vi "Example_DIO_DWG_Array.vi"() -> ()   [LabVIEW 2013]
uses:
  <vilib>/Signadyne/Wave/base/newFromArrayInteger.vi
  <vilib>/Signadyne/Wave/base/waveformLoadWave.vi
  Instance          11 29Saved   Example_DIO_DWG_Array .vi
panel:
  in  "Data":i32[][](array[numeric])=[[0], [1], [2], [3], [4], [5], [6], [7], [8], [9], [10], [11], [12], [13], [14], [15], [16], [17], [18], [19], [20], [21], [22], [23], [24], [25], [26], [27], [28], [29], [30], [31]]
  in  "End Line":i32=19
  in  "Start Line":i32=16
  in  "Slot":i32=5
  out "ConfigBus Status":errorcluster
  out "DirConfig":errorcluster
  out "Bus value":i64
  out "Close Status":errorcluster
  in  "Stop Loop":bool
  out "Open Status":errorcluster
  in  "Part Number":string="SD-PXE-DIO-H0002"
  # "Output&Input Bus"
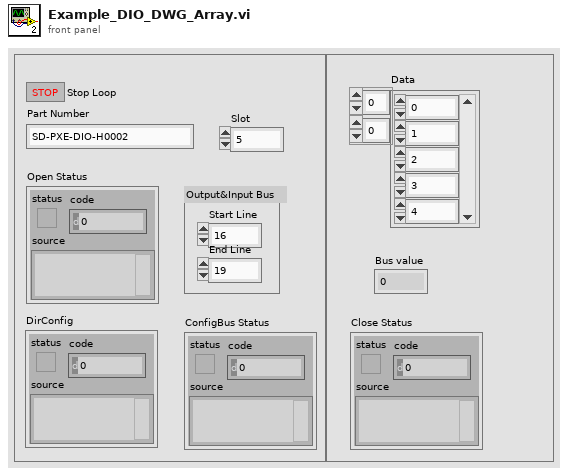
[diagram p1: front panel]
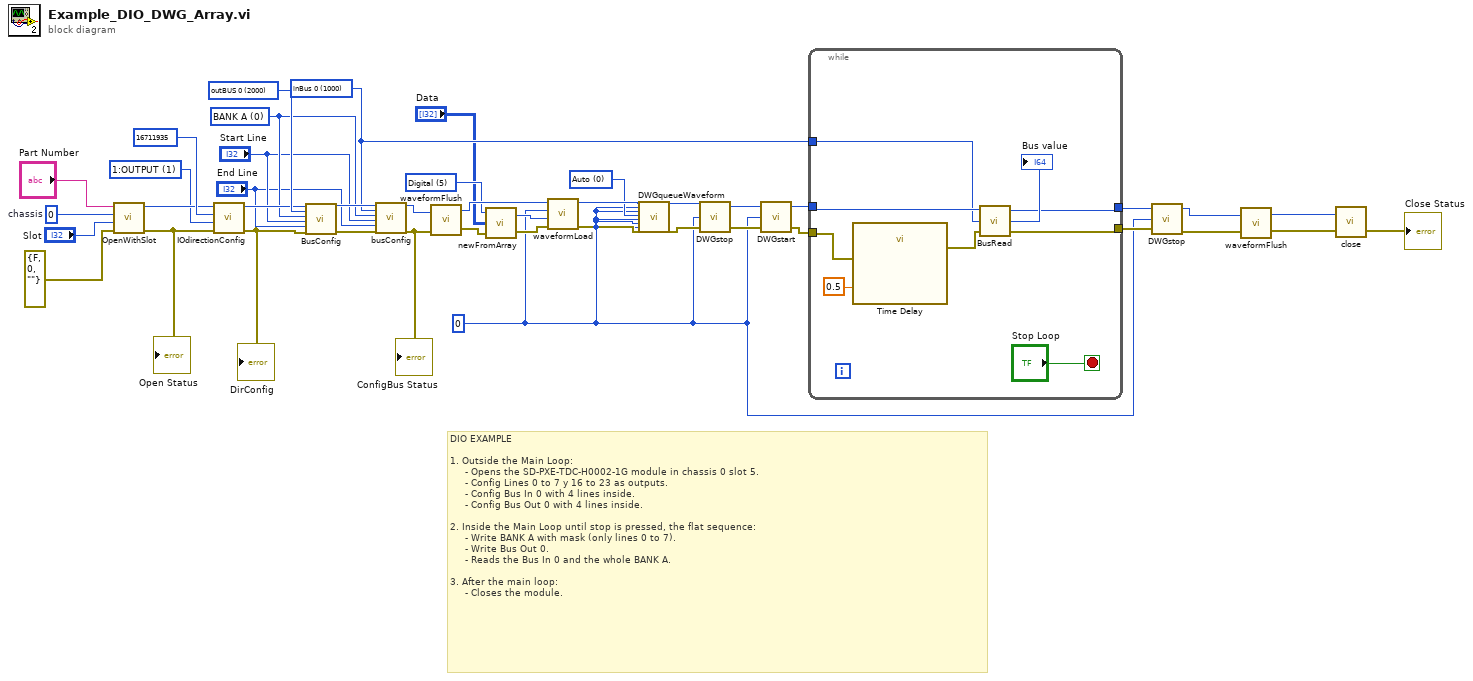
[diagram p0: block diagram]
diagram:
  w2 = 5 items=["Digital"=5] ("waveformType")
  w3 = 1000 items=["inBus 0"=1000, "inBus 1"=1001, "outBus 0"=2000, "outBus 1"=2001] ("nBus")
  w24 = 0 items=["Auto", "VI/HVI", "External"] ("triggerMode")
  w15 = 0 ("waveformNumber")
  w6 = 0 items=["BANK A"=0, "BANK B"=1, "BANK B:A"=3000] ("nPort")
  w35 = 2000 items=["inBus 0"=1000, "outBUS 0"=2000] ("nBus")
  w36 = u16 1 items=["0:INPUT", "1:OUTPUT"] ("direction")
  w40 = 0  # chassis
  # "DIO EXAMPLE\n\n1. Outside the Main Loop:\n     - Opens the SD-PXE-TDC-H0002-1G module in chassis 0 slot 5.\n     - Config Lines 0 to 7 y 16 to 23 as outputs.\n     - Config Bus In 0 with 4 lines inside.\n     - Config Bus Out 0 with 4 lines inside.\n\n2. Inside the Main Loop until stop is pressed, the flat sequence:\n     - Write BANK A with mask (only lines 0 to 7).\n     - Write Bus Out 0.\n     - Reads the Bus In 0 and the whole BANK A.\n\n3. After the main loop:\n     - Closes the module."
  n1 = call <vilib>:"OpenWithSlot.vi"("errorIn"=errorcluster {"status"=FALSE, "code"=0, "source"=""}, "nSlot"="Slot", "nChassis"=w40, "partNumber"="Part Number") -> ("errorOut"=w39:errorcluster, "moduleID"=w37:i32)  [unwired: 2 in]
  "Open Status" <- w39
  n2 = call <vilib>:"IOdirectionConfig.vi"("errorIn"=w39, "direction"=w36, "lineMask"=i64 16711935, "moduleID"=w37) -> ("errorOut"=w32:errorcluster, "moduleIDOut"=w31:i32)  [unwired: 2 in]
  "DirConfig" <- w32
  n3 = call <vilib>:"BusConfig.vi"("moduleID"=w31, "nBus"=w35, "port"=w6, "start"="Start Line", "end"="End Line", "errorIn"=w32) -> ("moduleIDOut"=w7:i32, "errorOut"=w8:errorcluster)  [unwired: 12 in]
  n4 = call <vilib>:"busConfig.vi"("moduleID"=w7, "nBus"=w3, "port"=w6, "start"="Start Line", "end"="End Line", "errorIn"=w8) -> ("moduleIDOut"=w10:i32, "errorOut"=w9:errorcluster)  [unwired: 12 in]
  "ConfigBus Status" <- w9
  n5 = call <vilib>:"waveformFlush.vi"("errorIn"=w9, "moduleID"=w10) -> ("errorOut"=w27:errorcluster, "moduleIDOut"=w28:i32)
  n6 = call-poly <vilib>:"newFromArray.vi"("errorIn"=w27, "waveformData"="Data", "waveformType"=w2) -> ("errorOut"=w30:errorcluster, "waveformID"=w29:i32)
  n7 = call-poly <vilib>:"waveformLoad.vi"("errorIn"=w30, "waveformID"=w29, "waveformNumber"=w15, "moduleID"=w28) -> ("errorOut"=w25:errorcluster, "moduleIDOut"=w26:i32)  [unwired: 5 in, 1 out]
  n8 = call <vilib>:"DWGqueueWaveform.vi"("moduleID"=w26, "DWG"=w15, "waveformNumber"=w15, "triggerMode"=w24, "startDelay"=w15, "cycles"=w15, "prescaler"=w15, "errorIn"=w25) -> ("moduleIDOut"=w22:i32, "errorOut"=w23:errorcluster)  [unwired: 18 in]
  n9 = call <vilib>:"DWGstop.vi"("errorIn"=w23, "DWG"=w15, "moduleID"=w22) -> ("errorOut"=w21:errorcluster, "moduleIDOut"=w20:i32)  [unwired: 1 in]
  n10 = call <vilib>:"DWGstart.vi"("errorIn"=w21, "DWG"=w15, "moduleID"=w20) -> ("errorOut"=w19:errorcluster, "moduleIDOut"=w18:i32)  [unwired: 1 in]
  n11 = while {
    tunnel: [w44] -> w16
    tunnel: [w45] -> w17
    tunnel: w18 -> [w46]
    tunnel: w19 -> [w47]
    tunnel: w3 -> [w43]
    stop <- "Stop Loop" stop-if-true
    n12 = call "Time Delay"("error in (no error)"=w47, "Delay Time (s)"=0.5) -> ("error out"=w49:errorcluster)  [unwired: 9 in]
    n13 = call <vilib>:"BusRead.vi"("errorIn"=w49, "inBus"=w43, "moduleID"=w46) -> ("errorOut"=w45:errorcluster, "portValue"=→"Bus value":i64, "moduleIDOut"=w44:i32)
  }
  n14 = call <vilib>:"DWGstop.vi"("errorIn"=w17, "DWG"=w15, "moduleID"=w16) -> ("errorOut"=w11:errorcluster, "moduleIDOut"=w12:i32)  [unwired: 1 in]
  n15 = call <vilib>:"waveformFlush.vi"("errorIn"=w11, "moduleID"=w12) -> ("errorOut"=w14:errorcluster, "moduleIDOut"=w13:i32)
  n16 = call <vilib>:"close.vi"("errorIn"=w14, "moduleID"=w13) -> ("errorOut"=→"Close Status":errorcluster)  [unwired: 1 in]
